vi "ProgramInitial.vi"(8 "error in (no error)":errorcluster, 11 "RealWorkActor in":refnum<class "RealWorkActor.lvclass">) -> (0 "error out":errorcluster, 3 "RealWorkActor out":refnum<class "RealWorkActor.lvclass">)   [LabVIEW 2014, in "RealWorkActor.lvlib" / "RealWorkActor.lvclass"]
uses:
  RealWorkActor.lvclass
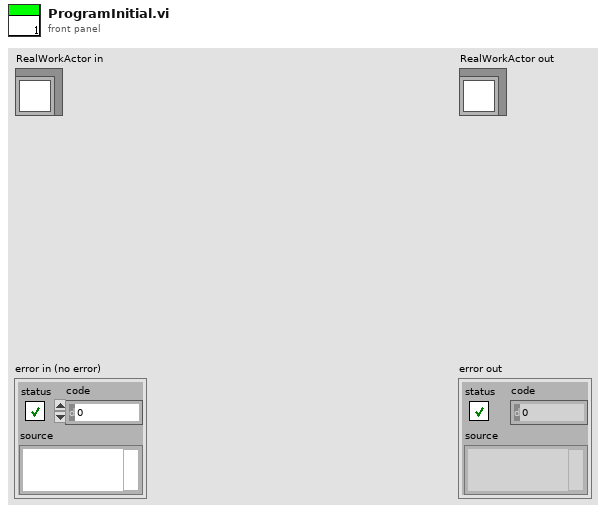
[diagram p1: front panel]
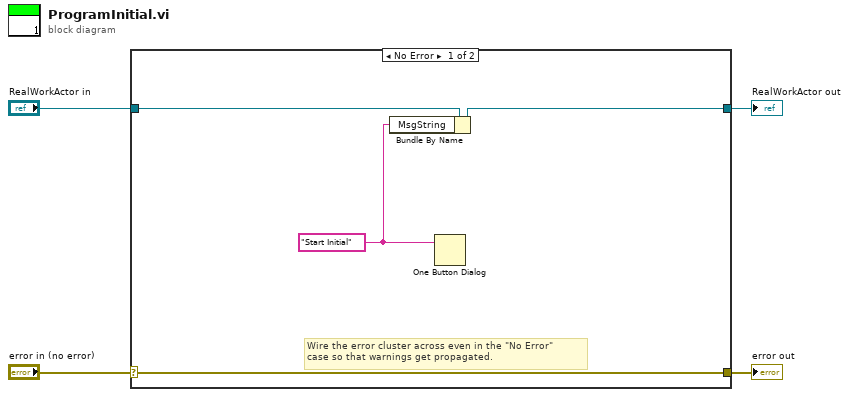
[diagram p0: block diagram]
diagram:
  n1 = case shown="No Error" "error in (no error)" {
    selector: "error in (no error)" -> [w7 w10]
    tunnel: [w7 w10] -> w3
    tunnel: [w6 w9] -> w1
    tunnel: "RealWorkActor in" -> [w8 w9]
    frame No Error {
      w5 = "Start Initial"
      # "Wire the error cluster across even in the \"No Error\"\ncase so that warnings get propagated."
      n2 = Bundle By Name(cluster=w8, "MsgString"=w5) -> (w6:refnum<class "RealWorkActor.lvclass">)
      n3 = One Button Dialog(message=w5) -> ()  [unwired: 1 in, 1 out]
    }
    frame Error {
    }
  }
  "error out" <- w3
  "RealWorkActor out" <- w1
